vi "PI_AreaScan_Prepare.vi"(0 "System":i32 min=0 max=3 step=1, 1 "Laser":string="1", 2 "Axis":string="xy", 3 "da":dbl min=-100.0 max=100.0, 4 "db":dbl min=-100.0 max=100.0, 5 "error in (no error)":errorcluster caption="Fehler (Eingang, kein Fehler)", 6 "a0":dbl=98.0 min=-98.0 max=98.0 step=0.01, 8 "b0":dbl min=-100.0 max=100.0 step=0.01, 9 "Resolution":dbl=0.01 min=0.01 max=2.0 step=0.01, 10 "c0":dbl min=-100.0 max=100.0, 11 "Pixel time":dbl) -> (14 "Tacq":dbl, 15 "TrigStartTo":dbl, 16 "TrigStopTo":dbl, 17 "TrigStartFrom":dbl, 18 "TrigStopFrom":dbl, 19 "error out":errorcluster caption="Fehler (Ausgang)")   [LabVIEW 2011]
panel:
  out "slow axis":i32
  out "fast axis":i32
  out "Accelaration":i32
  out "ttp":i32
  out "Scan lines":dbl
  out "Colors":i32
  out "Start position":dbl[](array[numeric])
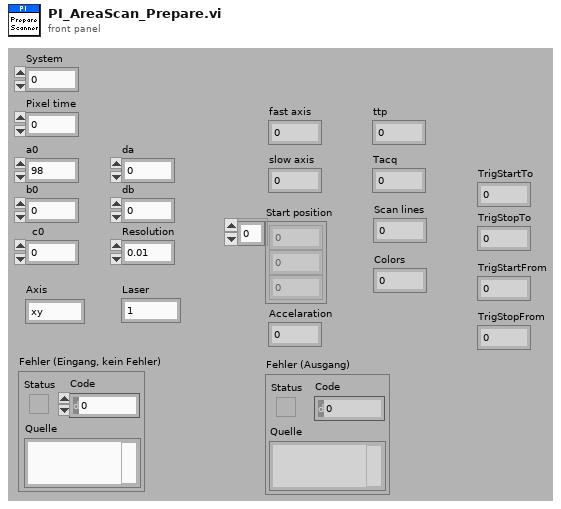
[diagram p1: front panel]
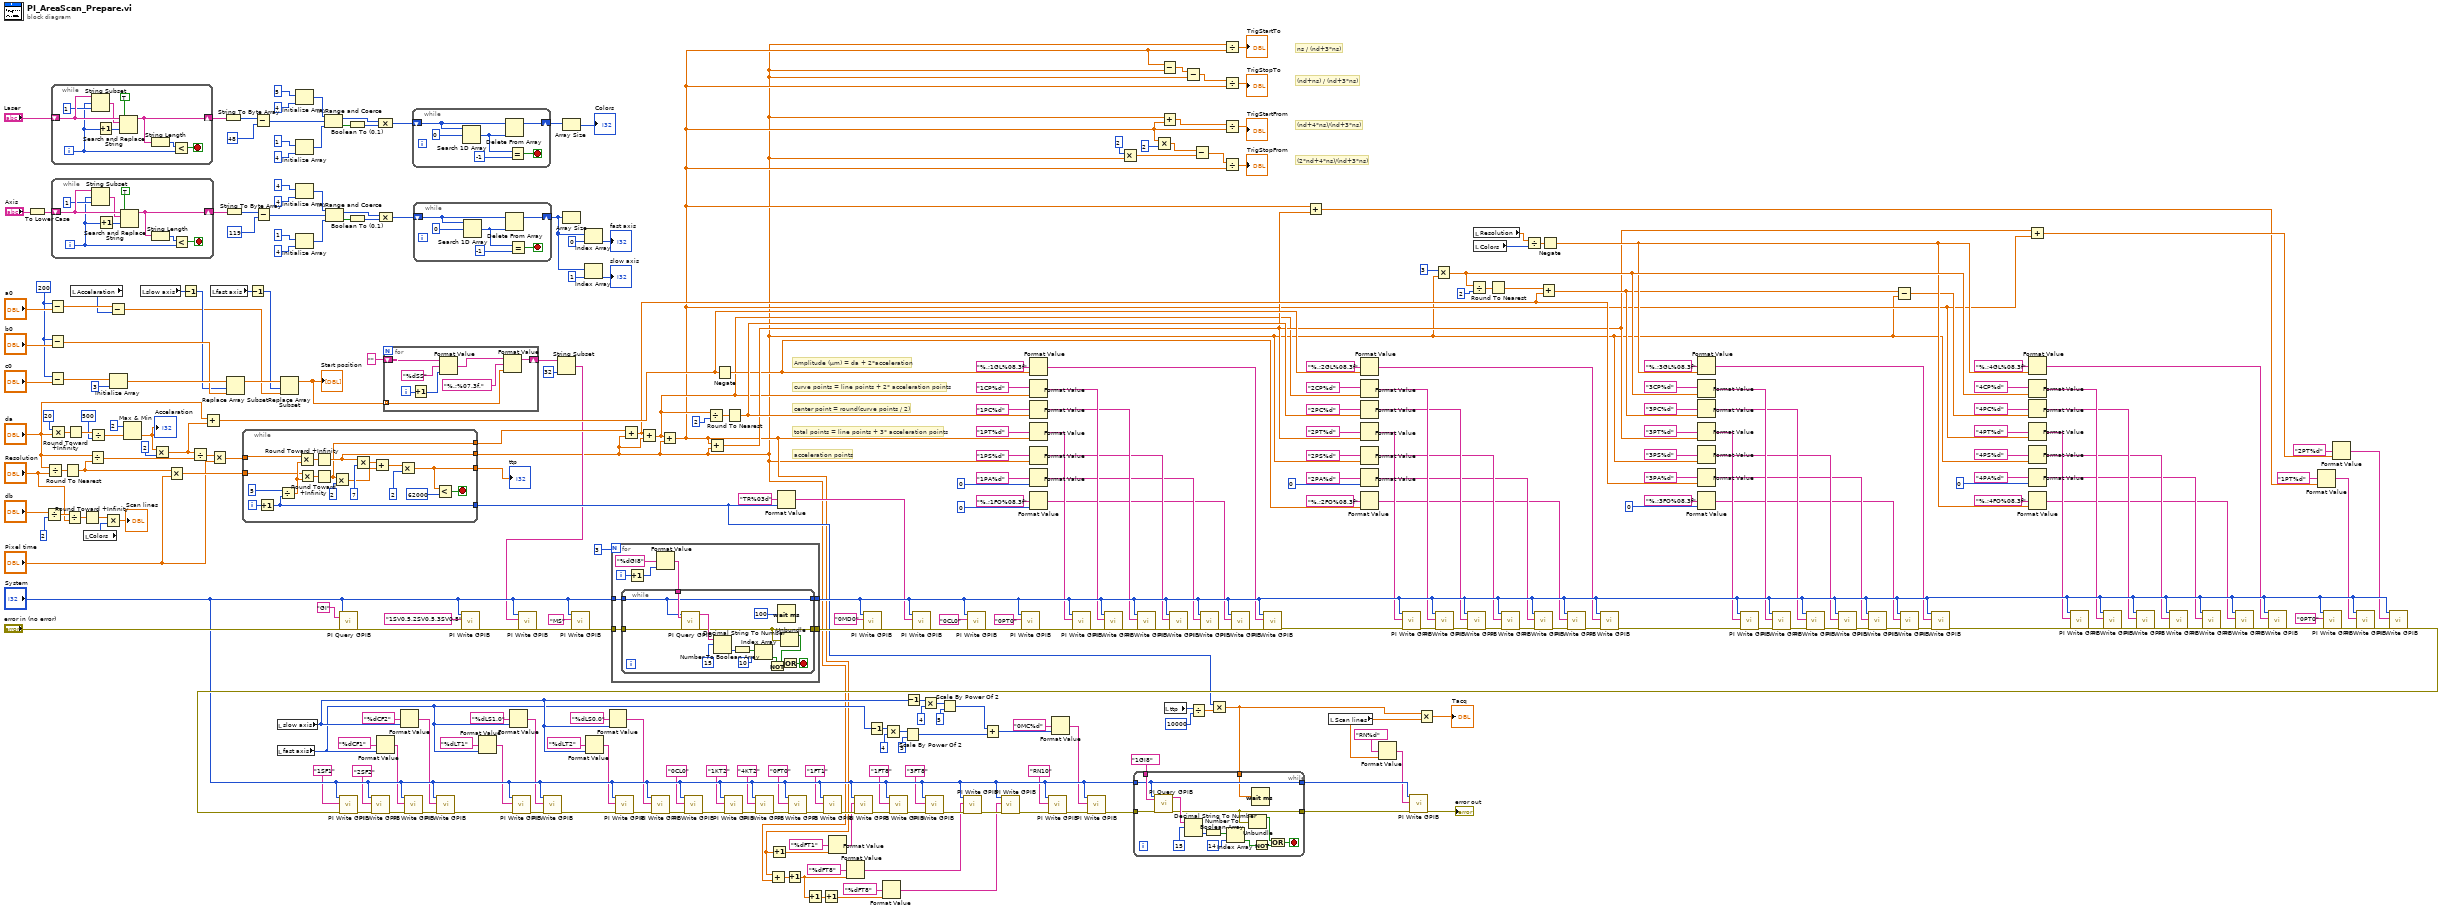
[diagram p0: block diagram]
diagram:
  w285 = 200
  # "(2*nd+4*ns)/(nd+3*ns)"
  # "(nd+4*ns)/(nd+3*ns)"
  # "(nd+ns) / (nd+3*ns)"
  # "ns / (nd+3*ns)"
  # "acceleration points"
  # "total points = line points + 3* acceleration points"
  # "center point = round(curve points / 2)"
  # "curve points = line points + 2* acceleration points"
  # "Amplitude (µm) = da + 2*acceleration"
  n1 = To Lower Case(string="Axis") -> (all lower case string=w289:string)
  n2 = Divide(x="db", y=2) -> (x/y=w263:dbl)
  n3 = Divide(x="da", y="Resolution") -> (x/y=w265:dbl)
  n4 = Subtract(x=w285, y="a0") -> (x-y=w268:dbl)
  n5 = Subtract(x=w285, y="b0") -> (x-y=w280:dbl)
  n6 = Subtract(x=w285, y="c0") -> (x-y=w282:dbl)
  n7 = Multiply(x=20, y="da") -> (x*y=w273:dbl)
  n8 = while {
    shift-right: [w325] -> w311
    shift-left: "Laser" -> [w329]
    i -> [w321]
    stop <- w324 stop-if-true
    n9 = String Subset(string=w329, offset (0)=w321, length (rest)=1) -> (substring=w327:string)
    n10 = Increment(x=w321) -> (x+1=w322:i32)
    n11 = Search and Replace String(replace all?=TRUE, input string=w329, search string=w327, offset=w322) -> (result string=w325:string)  [unwired: 4 in, 3 out]
    n12 = String Length(string=w325) -> (length=w323:i32)
    n13 = Less?(x=w323, y=w321) -> (x < y?=w324:bool)
  }
  n14 = while {
    shift-right: [w334] -> w295
    shift-left: w289 -> [w338]
    i -> [w330]
    stop <- w333 stop-if-true
    n15 = String Subset(string=w338, offset (0)=w330, length (rest)=1) -> (substring=w336:string)
    n16 = Increment(x=w330) -> (x+1=w331:i32)
    n17 = Search and Replace String(replace all?=TRUE, input string=w338, search string=w336, offset=w331) -> (result string=w334:string)  [unwired: 4 in, 3 out]
    n18 = String Length(string=w334) -> (length=w332:i32)
    n19 = Less?(x=w332, y=w330) -> (x < y?=w333:bool)
  }
  n20 = Round To Nearest(number=w265) -> (nearest integer value=w250:dbl)
  n21 = Divide(x=w263, y="Resolution") -> (x/y=w256:dbl)
  n22 = Round Toward +Infinity(x=w273) -> (ceil(x): smallest int >= x=w272:dbl)
  n23 = local read "Accelaration"() -> (w266:i32)
  n24 = Round Toward +Infinity(x=w256) -> (ceil(x): smallest int >= x=w257:dbl)
  n25 = local read "Colors"() -> (w259:i32)
  n26 = Divide(x="da", y=w250) -> (x/y=w249:dbl)
  n27 = Divide(x=w272, y=500) -> (x/y=w270:dbl)
  n28 = Multiply(x=w257, y=w259) -> (x*y=→"Scan lines":dbl)
  n29 = Subtract(x=w268, y=w266) -> (x-y=w267:dbl)
  n30 = Initialize Array(w282, 3) -> (w281:dbl[])
  n31 = Max & Min(x=2, y=w270) -> (min(x,y)=w211:dbl)  [unwired: 1 out]
  "Accelaration" <- w211
  n32 = local read "slow axis"() -> (w131:i32)
  n33 = Multiply(x=w211, y=2) -> (x*y=w220:dbl)
  n34 = Multiply(x=w250, y="Pixel time") -> (x*y=w255:dbl)
  n35 = Decrement(x=w131) -> (x-1=w277:i32)
  n36 = Divide(x=w220, y=w249) -> (x/y=w251:dbl)
  n37 = Add(x="da", y=w220) -> (x+y=w194:dbl)
  n38 = local read "fast axis"() -> (w132:i32)
  n39 = Multiply(x=w251, y="Pixel time") -> (x*y=w253:dbl)
  n40 = String To Byte Array(string=w311) -> (unsigned byte array=w313:u8[])
  n41 = String To Byte Array(string=w295) -> (unsigned byte array=w297:u8[])
  n42 = Replace Array Subset(array=w281, new element=w280, index=w277) -> (w278:dbl[])
  n43 = while {
    tunnel: w255 -> [w354]
    tunnel: w253 -> [w353]
    tunnel: [w342] -> w252
    tunnel: [w341] -> w90
    tunnel: [w340] -> w4
    tunnel: [w339] -> w225
    i -> [w357]
    stop <- w343 stop-if-true
    n44 = Increment(x=w357) -> (x+1=w341:i32)
    n45 = Divide(x=5, y=w341) -> (x/y=w355:dbl)
    n46 = Multiply(x=w353, y=w355) -> (x*y=w352:dbl)
    n47 = Multiply(x=w354, y=w355) -> (x*y=w351:dbl)
    n48 = Round Toward +Infinity(x=w352) -> (ceil(x): smallest int >= x=w340:dbl)
    n49 = Round Toward +Infinity(x=w351) -> (ceil(x): smallest int >= x=w339:dbl)
    n50 = Multiply(x=w339, y=2) -> (x*y=w347:dbl)
    n51 = Multiply(x=w340, y=7) -> (x*y=w348:dbl)
    n52 = Add(x=w348, y=w347) -> (x+y=w346:dbl)
    n53 = Multiply(x=w346, y=2) -> (x*y=w342:dbl)
    n54 = Less?(x=w342, y=62000) -> (x < y?=w343:bool)
  }
  "ttp" <- w252
  n55 = Decrement(x=w132) -> (x-1=w276:i32)
  n56 = Subtract(x=w313, y=48) -> (x-y=w310:i32[])
  n57 = Subtract(x=w297, y=119) -> (x-y=w294:i32[])
  n58 = local read "slow axis"() -> (w105:i32)
  n59 = local read "fast axis"() -> (w96:i32)
  n60 = Replace Array Subset(array=w278, new element=w267, index=w276) -> (w244:dbl[])
  "Start position" <- w244
  n61 = Initialize Array(5, 4) -> (w318:i32[])
  n62 = Initialize Array(1, 4) -> (w315:i32[])
  n63 = Initialize Array(4, 4) -> (w302:i32[])
  n64 = Initialize Array(1, 4) -> (w299:i32[])
  n65 = In Range and Coerce(upper limit=w318, x=w310, lower limit=w315) -> (coerced(x)=w307:i32[], In Range?=w314:bool[])
  n66 = In Range and Coerce(upper limit=w302, x=w294, lower limit=w299) -> (coerced(x)=w291:i32[], In Range?=w298:bool[])
  n67 = call "PI Query GPIB.vi"("System no."="System", "String to send"="GI", "error in"="error in (no error)") -> ("error out"=w246:errorcluster)  [unwired: 14 in, 2 out]
  n68 = Boolean To (0,1)(Boolean=w314) -> (0, 1=w308:i16[])
  n69 = Boolean To (0,1)(Boolean=w298) -> (0, 1=w292:i16[])
  n70 = Format Value(format string="%dCF1", value (0)=w96) -> (output string=w28:string)  [unwired: 1 in]
  n71 = Compound Arithmetic op=MULTIPLY(w307, w308) -> (w309:i32[])
  n72 = Compound Arithmetic op=MULTIPLY(w291, w292) -> (w293:i32[])
  n73 = for {
    shift-right: [w363] -> w243
    shift-left: "" -> [w365]
    tunnel: w244 -> [w358] mode=indexing
    i -> [w360]
    n74 = Increment(x=w360) -> (x+1=w359:i32)
    n75 = Format Value(string ("")=w365, format string="%dSS", value (0)=w359) -> (output string=w364:string)
    n76 = Format Value(string ("")=w364, format string="%.;%07.3f,", value (0)=w358) -> (output string=w363:string)
  }
  n77 = Format Value(format string="%dCF2", value (0)=w105) -> (output string=w27:string)  [unwired: 1 in]
  n78 = while {
    shift-right: [w368] -> w306
    shift-left: w309 -> [w366]
    stop <- w369 stop-if-true
    n79 = Search 1D Array(1D array=w366, element=0) -> (index of element=w370:i32)  [unwired: 1 in]
    n80 = Delete From Array(array=w366, index=w370) -> (array with subset deleted=w368:i32[])  [unwired: 1 in, 1 out]
    n81 = Equal?(x=w370, y=-1) -> (x = y?=w369:bool)
  }
  n82 = while {
    shift-right: [w374] -> w275
    shift-left: w293 -> [w372]
    stop <- w375 stop-if-true
    n83 = Search 1D Array(1D array=w372, element=0) -> (index of element=w376:i32)  [unwired: 1 in]
    n84 = Delete From Array(array=w372, index=w376) -> (array with subset deleted=w374:i32[])  [unwired: 1 in, 1 out]
    n85 = Equal?(x=w376, y=-1) -> (x = y?=w375:bool)
  }
  n86 = call "PI Write GPIB.vi"("System no."="System", "String to send"="1SV0.5,2SV0.5,3SV0.5", "error in"=w246) -> ("error out"=w241:errorcluster)  [unwired: 16 in]
  n87 = Format Value(format string="%dLT1", value (0)=w96) -> (output string=w26:string)  [unwired: 1 in]
  n88 = Format Value(format string="%dLS1.0", value (0)=w96) -> (output string=w25:string)  [unwired: 1 in]
  n89 = String Subset(string=w243, length (rest)=32) -> (substring=w67:string)  [unwired: 1 in]
  n90 = call "PI Write GPIB.vi"("System no."="System", "String to send"=w67, "error in"=w241) -> ("error out"=w240:errorcluster)  [unwired: 16 in]
  n91 = Array Size(array=w306) -> (size(s)=→"Colors":i32)
  n92 = Array Size(array=w275) -> ()  [unwired: 1 out]
  n93 = call "PI Write GPIB.vi"("System no."="System", "String to send"="MS", "error in"=w240) -> ("error out"=w239:errorcluster)  [unwired: 16 in]
  n94 = Index Array(array=w275, index=0) -> (element=→"fast axis":i32)
  n95 = Index Array(array=w275, index=1) -> (element=→"slow axis":i32)
  n96 = Format Value(format string="%dLT2", value (0)=w105) -> (output string=w24:string)  [unwired: 1 in]
  n97 = Format Value(format string="%dLS0.0", value (0)=w105) -> (output string=w23:string)  [unwired: 1 in]
  n98 = for {
    N: 3 -> [_]
    tunnel: w239 -> [w381]
    tunnel: "System" -> [w380]
    tunnel: [w379] -> w237
    tunnel: [w378] -> w150
    i -> [w385]
    n99 = Increment(x=w385) -> (x+1=w384:i32)
    n100 = Format Value(format string="%dGI8", value (0)=w384) -> (output string=w382:string)  [unwired: 1 in]
    n101 = while {
      tunnel: w382 -> [w399]
      tunnel: w381 -> [w398]
      tunnel: w380 -> [w394]
      tunnel: [w393] -> w379
      tunnel: [w394] -> w378
      stop <- w388 stop-if-true
      n102 = call "PI Query GPIB.vi"("System no."=w394, "String to send"=w399, "error in"=w398) -> ("String read"=w396:string, "error out"=w393:errorcluster)  [unwired: 14 in, 1 out]
      n103 = Decimal String To Number(string=w396, offset=15) -> (number=w395:i32)  [unwired: 1 in, 1 out]
      n104 = Number To Boolean Array(number=w395) -> (Boolean array=w390:bool[])
      n105 = Index Array(array=w390, index=10) -> (element=w389:bool)
      n106 = Not(x=w389) -> (.not. x?=w386:bool)
      n107 = Wait (ms)(milliseconds to wait=100) -> ()  [unwired: 1 out]
      n108 = Unbundle(w393) -> ("status"=w392:bool)  [unwired: 2 out]
      n109 = Or(x=w392, y=w386) -> (x .or. y?=w388:bool)
    }
  }
  n110 = Add(x=w225, y=w4) -> (x+y=w159:dbl)
  n111 = Add(x=w159, y=w4) -> (x+y=w78:dbl)
  n112 = Add(x=w78, y=w4) -> (x+y=w5:dbl)
  n113 = Divide(x=w78, y=2) -> (x/y=w223:dbl)
  n114 = Add(x=w5, y=w4) -> (x+y=w144:dbl)
  n115 = Negate(x=w194) -> (-x=w116:dbl)
  n116 = Round To Nearest(number=w223) -> (nearest integer value=w195:dbl)
  n117 = Add(x=w5, y=w4) -> (x+y=w3:dbl)
  n118 = Increment(x=w5) -> (x+1=w117:dbl)
  n119 = Format Value(format string="TR%03d", value (0)=w90) -> (output string=w64:string)  [unwired: 1 in]
  n120 = Increment(x=w3) -> (x+1=w1:dbl)
  n121 = Increment(x=w1) -> (x+1=w2:dbl)
  n122 = Increment(x=w2) -> (x+1=w8:dbl)
  n123 = Format Value(format string="%dFT1", value (0)=w117) -> (output string=w17:string)  [unwired: 1 in]
  n124 = Format Value(format string="%dFT8", value (0)=w1) -> (output string=w7:string)  [unwired: 1 in]
  n125 = call "PI Write GPIB.vi"("System no."=w150, "String to send"="0MD0", "error in"=w237) -> ("error out"=w236:errorcluster)  [unwired: 16 in]
  n126 = Decrement(x=w96) -> (x-1=w101:i32)
  n127 = Format Value(format string="%dFT8", value (0)=w8) -> (output string=w6:string)  [unwired: 1 in]
  n128 = Multiply(x=w101, y=4) -> (x*y=w103:i32)
  n129 = Scale By Power Of 2(n=w103, x=u8 5) -> (x*2^n=w99:u8)
  n130 = Decrement(x=w105) -> (x-1=w106:i32)
  n131 = call "PI Write GPIB.vi"("System no."=w150, "String to send"=w64, "error in"=w236) -> ("error out"=w234:errorcluster)  [unwired: 16 in]
  n132 = Multiply(x=w106, y=4) -> (x*y=w108:i32)
  n133 = Scale By Power Of 2(n=w108, x=u8 5) -> (x*2^n=w100:u8)
  n134 = call "PI Write GPIB.vi"("System no."=w150, "String to send"="0CL0", "error in"=w234) -> ("error out"=w233:errorcluster)  [unwired: 16 in]
  n135 = Add(x=w100, y=w99) -> (x+y=w98:u8)
  n136 = call "PI Write GPIB.vi"("System no."=w150, "String to send"="0PT0", "error in"=w233) -> ("error out"=w218:errorcluster)  [unwired: 16 in]
  n137 = Format Value(format string="%.;1GL%08.3f", value (0)=w116) -> (output string=w56:string)  [unwired: 1 in]
  n138 = Format Value(format string="1CP%d", value (0)=w78) -> (output string=w61:string)  [unwired: 1 in]
  n139 = Format Value(format string="1PC%d", value (0)=w195) -> (output string=w60:string)  [unwired: 1 in]
  n140 = Format Value(format string="1PT%d", value (0)=w5) -> (output string=w62:string)  [unwired: 1 in]
  n141 = Format Value(format string="1PS%d", value (0)=w4) -> (output string=w59:string)  [unwired: 1 in]
  n142 = Format Value(format string="1PA%d", value (0)=0) -> (output string=w58:string)  [unwired: 1 in]
  n143 = Format Value(format string="%.;1FO%08.3f", value (0)=0) -> (output string=w57:string)  [unwired: 1 in]
  n144 = Format Value(format string="0MC%d", value (0)=w98) -> (output string=w13:string)  [unwired: 1 in]
  n145 = call "PI Write GPIB.vi"("System no."=w150, "String to send"=w62, "error in"=w218) -> ("error out"=w212:errorcluster)  [unwired: 16 in]
  n146 = call "PI Write GPIB.vi"("System no."=w150, "String to send"=w61, "error in"=w212) -> ("error out"=w217:errorcluster)  [unwired: 16 in]
  n147 = Multiply(x=2, y=w4) -> (x*y=w70:dbl)
  n148 = call "PI Write GPIB.vi"("System no."=w150, "String to send"=w60, "error in"=w217) -> ("error out"=w216:errorcluster)  [unwired: 16 in]
  n149 = Multiply(x=w5, y=2) -> (x*y=w69:dbl)
  n150 = Subtract(x=w5, y=w4) -> (x-y=w74:dbl)
  n151 = Add(x=w4, y=w5) -> (x+y=w75:dbl)
  n152 = local read "ttp"() -> (w93:i32)
  n153 = call "PI Write GPIB.vi"("System no."=w150, "String to send"=w59, "error in"=w216) -> ("error out"=w215:errorcluster)  [unwired: 16 in]
  n154 = Subtract(x=w74, y=w4) -> (x-y=w73:dbl)
  n155 = Divide(x=w93, y=10000) -> (x/y=w91:dbl)
  n156 = Subtract(x=w69, y=w70) -> (x-y=w68:dbl)
  n157 = call "PI Write GPIB.vi"("System no."=w150, "String to send"=w58, "error in"=w215) -> ("error out"=w214:errorcluster)  [unwired: 16 in]
  n158 = Multiply(x=w90, y=w91) -> (x*y=w86:dbl)
  n159 = Divide(x=w4, y=w5) -> (x/y=→"TrigStartTo":dbl)
  n160 = Divide(x=w73, y=w5) -> (x/y=→"TrigStopTo":dbl)
  n161 = Divide(x=w75, y=w5) -> (x/y=→"TrigStartFrom":dbl)
  n162 = Divide(x=w68, y=w5) -> (x/y=→"TrigStopFrom":dbl)
  n163 = call "PI Write GPIB.vi"("System no."=w150, "String to send"=w57, "error in"=w214) -> ("error out"=w213:errorcluster)  [unwired: 16 in]
  n164 = call "PI Write GPIB.vi"("System no."=w150, "String to send"=w56, "error in"=w213) -> ("error out"=w204:errorcluster)  [unwired: 16 in]
  n165 = Add(x=w5, y=w144) -> (x+y=w83:dbl)
  n166 = local read "Scan lines"() -> (w87:dbl)
  n167 = Format Value(format string="%.;2GL%08.3f", value (0)=w194) -> (output string=w49:string)  [unwired: 1 in]
  n168 = Format Value(format string="2CP%d", value (0)=w78) -> (output string=w54:string)  [unwired: 1 in]
  n169 = Format Value(format string="2PC%d", value (0)=w195) -> (output string=w53:string)  [unwired: 1 in]
  n170 = Format Value(format string="2PT%d", value (0)=w144) -> (output string=w55:string)  [unwired: 1 in]
  n171 = Format Value(format string="2PS%d", value (0)=w4) -> (output string=w52:string)  [unwired: 1 in]
  n172 = Format Value(format string="2PA%d", value (0)=0) -> (output string=w51:string)  [unwired: 1 in]
  n173 = Format Value(format string="%.;2FO%08.3f", value (0)=w116) -> (output string=w50:string)  [unwired: 1 in]
  n174 = Format Value(format string="RN%d", value (0)=w87) -> (output string=w12:string)  [unwired: 1 in]
  n175 = call "PI Write GPIB.vi"("System no."=w150, "String to send"=w55, "error in"=w204) -> ("error out"=w205:errorcluster)  [unwired: 16 in]
  n176 = Multiply(x=w86, y=w87) -> (x*y=→"Tacq":dbl)
  n177 = Multiply(x=3, y=w4) -> (x*y=w155:dbl)
  n178 = call "PI Write GPIB.vi"("System no."=w150, "String to send"=w54, "error in"=w205) -> ("error out"=w210:errorcluster)  [unwired: 16 in]
  n179 = call "PI Write GPIB.vi"("System no."=w150, "String to send"=w53, "error in"=w210) -> ("error out"=w209:errorcluster)  [unwired: 16 in]
  n180 = Divide(x=w155, y=2) -> (x/y=w161:dbl)
  n181 = local read "Resolution"() -> (w158:dbl)
  n182 = local read "Colors"() -> (w157:i32)
  n183 = Round To Nearest(number=w161) -> (nearest integer value=w160:dbl)
  n184 = call "PI Write GPIB.vi"("System no."=w150, "String to send"=w52, "error in"=w209) -> ("error out"=w208:errorcluster)  [unwired: 16 in]
  n185 = Divide(x=w158, y=w157) -> (x/y=w156:dbl)
  n186 = call "PI Write GPIB.vi"("System no."=w150, "String to send"=w51, "error in"=w208) -> ("error out"=w207:errorcluster)  [unwired: 16 in]
  n187 = Add(x=w160, y=w159) -> (x+y=w152:dbl)
  n188 = Negate(x=w156) -> (-x=w154:dbl)
  n189 = call "PI Write GPIB.vi"("System no."=w150, "String to send"=w50, "error in"=w207) -> ("error out"=w206:errorcluster)  [unwired: 16 in]
  n190 = call "PI Write GPIB.vi"("System no."=w150, "String to send"=w49, "error in"=w206) -> ("error out"=w164:errorcluster)  [unwired: 16 in]
  n191 = Format Value(format string="%.;3GL%08.3f", value (0)=w154) -> (output string=w42:string)  [unwired: 1 in]
  n192 = Format Value(format string="3CP%d", value (0)=w155) -> (output string=w47:string)  [unwired: 1 in]
  n193 = Format Value(format string="3PC%d", value (0)=w152) -> (output string=w46:string)  [unwired: 1 in]
  n194 = Format Value(format string="3PT%d", value (0)=w144) -> (output string=w48:string)  [unwired: 1 in]
  n195 = Format Value(format string="3PS%d", value (0)=w4) -> (output string=w45:string)  [unwired: 1 in]
  n196 = Format Value(format string="3PA%d", value (0)=w159) -> (output string=w44:string)  [unwired: 1 in]
  n197 = Format Value(format string="%.;3FO%08.3f", value (0)=0) -> (output string=w43:string)  [unwired: 1 in]
  n198 = call "PI Write GPIB.vi"("System no."=w150, "String to send"=w48, "error in"=w164) -> ("error out"=w180:errorcluster)  [unwired: 16 in]
  n199 = call "PI Write GPIB.vi"("System no."=w150, "String to send"=w47, "error in"=w180) -> ("error out"=w185:errorcluster)  [unwired: 16 in]
  n200 = call "PI Write GPIB.vi"("System no."=w150, "String to send"=w46, "error in"=w185) -> ("error out"=w184:errorcluster)  [unwired: 16 in]
  n201 = call "PI Write GPIB.vi"("System no."=w150, "String to send"=w45, "error in"=w184) -> ("error out"=w183:errorcluster)  [unwired: 16 in]
  n202 = call "PI Write GPIB.vi"("System no."=w150, "String to send"=w44, "error in"=w183) -> ("error out"=w182:errorcluster)  [unwired: 16 in]
  n203 = Subtract(x=w152, y=w4) -> (x-y=w153:dbl)
  n204 = call "PI Write GPIB.vi"("System no."=w150, "String to send"=w43, "error in"=w182) -> ("error out"=w181:errorcluster)  [unwired: 16 in]
  n205 = call "PI Write GPIB.vi"("System no."=w150, "String to send"=w42, "error in"=w181) -> ("error out"=w173:errorcluster)  [unwired: 16 in]
  n206 = Add(x=w144, y=w5) -> (x+y=w145:dbl)
  n207 = Format Value(format string="%.;4GL%08.3f", value (0)=w154) -> (output string=w35:string)  [unwired: 1 in]
  n208 = Format Value(format string="4CP%d", value (0)=w155) -> (output string=w40:string)  [unwired: 1 in]
  n209 = Format Value(format string="4PC%d", value (0)=w153) -> (output string=w39:string)  [unwired: 1 in]
  n210 = Format Value(format string="4PT%d", value (0)=w5) -> (output string=w41:string)  [unwired: 1 in]
  n211 = Format Value(format string="4PS%d", value (0)=w4) -> (output string=w38:string)  [unwired: 1 in]
  n212 = Format Value(format string="4PA%d", value (0)=0) -> (output string=w37:string)  [unwired: 1 in]
  n213 = Format Value(format string="%.;4FO%08.3f", value (0)=w154) -> (output string=w36:string)  [unwired: 1 in]
  n214 = call "PI Write GPIB.vi"("System no."=w150, "String to send"=w41, "error in"=w173) -> ("error out"=w174:errorcluster)  [unwired: 16 in]
  n215 = call "PI Write GPIB.vi"("System no."=w150, "String to send"=w40, "error in"=w174) -> ("error out"=w179:errorcluster)  [unwired: 16 in]
  n216 = call "PI Write GPIB.vi"("System no."=w150, "String to send"=w39, "error in"=w179) -> ("error out"=w178:errorcluster)  [unwired: 16 in]
  n217 = call "PI Write GPIB.vi"("System no."=w150, "String to send"=w38, "error in"=w178) -> ("error out"=w177:errorcluster)  [unwired: 16 in]
  n218 = call "PI Write GPIB.vi"("System no."=w150, "String to send"=w37, "error in"=w177) -> ("error out"=w176:errorcluster)  [unwired: 16 in]
  n219 = call "PI Write GPIB.vi"("System no."=w150, "String to send"=w36, "error in"=w176) -> ("error out"=w175:errorcluster)  [unwired: 16 in]
  n220 = call "PI Write GPIB.vi"("System no."=w150, "String to send"=w35, "error in"=w175) -> ("error out"=w151:errorcluster)  [unwired: 16 in]
  n221 = Format Value(format string="1PT%d", value (0)=w83) -> (output string=w33:string)  [unwired: 1 in]
  n222 = call "PI Write GPIB.vi"("System no."=w150, "String to send"="0PT0", "error in"=w151) -> ("error out"=w149:errorcluster)  [unwired: 16 in]
  n223 = Format Value(format string="2PT%d", value (0)=w145) -> (output string=w32:string)  [unwired: 1 in]
  n224 = call "PI Write GPIB.vi"("System no."=w150, "String to send"=w33, "error in"=w149) -> ("error out"=w148:errorcluster)  [unwired: 16 in]
  n225 = call "PI Write GPIB.vi"("System no."=w150, "String to send"=w32, "error in"=w148) -> ("error out"=w137:errorcluster)  [unwired: 16 in]
  n226 = call "PI Write GPIB.vi"("System no."="System", "String to send"="1SF1", "error in"=w137) -> ("error out"=w138:errorcluster)  [unwired: 16 in]
  n227 = call "PI Write GPIB.vi"("System no."="System", "String to send"="2SF2", "error in"=w138) -> ("error out"=w143:errorcluster)  [unwired: 16 in]
  n228 = call "PI Write GPIB.vi"("System no."="System", "String to send"=w28, "error in"=w143) -> ("error out"=w142:errorcluster)  [unwired: 16 in]
  n229 = call "PI Write GPIB.vi"("System no."="System", "String to send"=w27, "error in"=w142) -> ("error out"=w141:errorcluster)  [unwired: 16 in]
  n230 = call "PI Write GPIB.vi"("System no."="System", "String to send"=w26, "error in"=w141) -> ("error out"=w140:errorcluster)  [unwired: 16 in]
  n231 = call "PI Write GPIB.vi"("System no."="System", "String to send"=w25, "error in"=w140) -> ("error out"=w139:errorcluster)  [unwired: 16 in]
  n232 = call "PI Write GPIB.vi"("System no."="System", "String to send"=w24, "error in"=w139) -> ("error out"=w125:errorcluster)  [unwired: 16 in]
  n233 = call "PI Write GPIB.vi"("System no."="System", "String to send"=w23, "error in"=w125) -> ("error out"=w126:errorcluster)  [unwired: 16 in]
  n234 = call "PI Write GPIB.vi"("System no."="System", "String to send"="0CL0", "error in"=w126) -> ("error out"=w122:errorcluster)  [unwired: 16 in]
  n235 = call "PI Write GPIB.vi"("System no."="System", "String to send"="1KT2", "error in"=w122) -> ("error out"=w123:errorcluster)  [unwired: 16 in]
  n236 = call "PI Write GPIB.vi"("System no."="System", "String to send"="4KT2", "error in"=w123) -> ("error out"=w124:errorcluster)  [unwired: 16 in]
  n237 = call "PI Write GPIB.vi"("System no."="System", "String to send"="0FT0", "error in"=w124) -> ("error out"=w119:errorcluster)  [unwired: 16 in]
  n238 = call "PI Write GPIB.vi"("System no."="System", "String to send"="1FT1", "error in"=w119) -> ("error out"=w120:errorcluster)  [unwired: 16 in]
  n239 = call "PI Write GPIB.vi"("System no."="System", "String to send"=w17, "error in"=w120) -> ("error out"=w121:errorcluster)  [unwired: 16 in]
  n240 = call "PI Write GPIB.vi"("System no."="System", "String to send"="1FT8", "error in"=w121) -> ("error out"=w115:errorcluster)  [unwired: 16 in]
  n241 = call "PI Write GPIB.vi"("System no."="System", "String to send"="3FT8", "error in"=w115) -> ("error out"=w114:errorcluster)  [unwired: 16 in]
  n242 = call "PI Write GPIB.vi"("System no."="System", "String to send"=w7, "error in"=w114) -> ("error out"=w113:errorcluster)  [unwired: 16 in]
  n243 = call "PI Write GPIB.vi"("System no."="System", "String to send"=w6, "error in"=w113) -> ("error out"=w111:errorcluster)  [unwired: 16 in]
  n244 = call "PI Write GPIB.vi"("System no."="System", "String to send"="RN10", "error in"=w111) -> ("error out"=w112:errorcluster)  [unwired: 16 in]
  n245 = call "PI Write GPIB.vi"("System no."="System", "String to send"=w13, "error in"=w112) -> ("error out"=w97:errorcluster)  [unwired: 16 in]
  n246 = while {
    tunnel: "1GI8" -> [w413]
    tunnel: w97 -> [w412]
    tunnel: "System" -> [w408]
    tunnel: [w403] -> w81
    tunnel: [w408] -> w82
    tunnel: w86 -> [w407]
    stop <- w404 stop-if-true
    n247 = call "PI Query GPIB.vi"("System no."=w408, "String to send"=w413, "error in"=w412) -> ("String read"=w410:string, "error out"=w403:errorcluster)  [unwired: 14 in, 1 out]
    n248 = Decimal String To Number(string=w410, offset=15) -> (number=w409:i32)  [unwired: 1 in, 1 out]
    n249 = Number To Boolean Array(number=w409) -> (Boolean array=w406:bool[])
    n250 = Index Array(array=w406, index=14) -> (element=w402:bool)
    n251 = Unbundle(w403) -> ("status"=w401:bool)  [unwired: 2 out]
    n252 = Wait (ms)(milliseconds to wait=w407) -> ()  [unwired: 1 out]
    n253 = Not(x=w402) -> (.not. x?=w400:bool)
    n254 = Or(x=w401, y=w400) -> (x .or. y?=w404:bool)
  }
  n255 = call "PI Write GPIB.vi"("System no."=w82, "String to send"=w12, "error in"=w81) -> ("error out"=→"error out":errorcluster)  [unwired: 16 in]
